vi "LV Exp7.vi"() -> ()   [LabVIEW 2009]
uses:
  <vilib>/NXT/Block Support/NXT_InputPort.ctl
  <vilib>/NXT/Dual Mode Library/Waits/Wait_Num(msec).vi
  <vilib>/NXT/Dual Mode Library/Display/drawText.vi
panel:
  out "Detected":bool
  # "HiTechnic Experimenter's Kit\n\n                        Experiment 7 - Magnetic Switch\nThis program reads the status of the Hall Effect Sensor on B0\nto determine if a magnetic field is presen and if it is present\nthe LED on B4 is truned on.\n\nSee Experimenter's Kit Handbook for the SuperPro for\nmore information or go to www.hitechnic.com. \n\n(c) HiTechnic 2011"
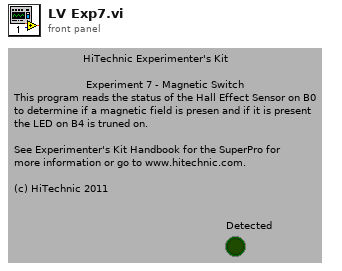
[diagram p1: front panel]
types:
  T1 = typedef "NXT_InputPort.ctl" = u8
  T2 = typedef "LVHSConnector.ctl" = cluster{"error":errorcluster, "address":string, "NXT #":i32, "Show Error":bool, "Connection":u16}
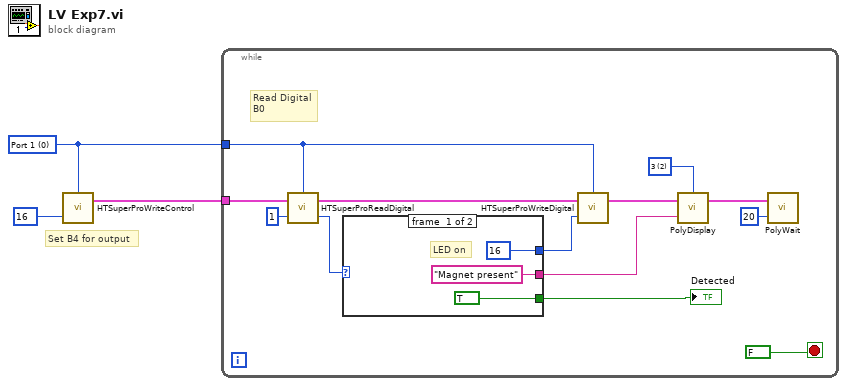
[diagram p0: block diagram]
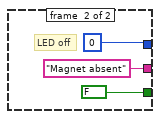
[diagram p2: hidden frame]
diagram:
  w1 = T1 0 items=["Port 1", "Port 2", "Port 3", "Port 4"] ("Port")
  # "Set B4 for output"
  n1 = call "HTSuperProWriteControl.vi"("Digital Value"=u8 16, "Port"=w1) -> ("NXT"=w2:T2)  [unwired: 3 in]
  n2 = while {
    tunnel: w2 -> [w13]
    tunnel: w1 -> [w10]
    stop <- FALSE stop-if-true
    w4 = i16 2 items=["1", "2", "3", "4", "5", "6", "7", "8"] ("Line")
    # "Read Digital\nB0"
    n3 = call "HTSuperProReadDigital.vi"("Mask"=u8 1, "NXT"=w13, "Port"=w10) -> ("Digital Value"=w12:u8, "NXT"=w11:T2)  [unwired: 1 in]
    n4 = case shown="1" w12 {
      tunnel: ["Magnet present" "Magnet absent"] -> w7
      tunnel: [TRUE FALSE] -> w15
      tunnel: [u8 16 u8 0] -> w9
      frame #0 {
        # "LED on"
      }
      frame #1 {
        # "LED off"
      }
    }
    "Detected" <- w15
    n5 = call "HTSuperProWriteDigital.vi"("Digital Value"=w9, "NXT"=w11, "Port"=w10) -> ("NXT"=w8:T2)  [unwired: 2 in]
    n6 = call-poly <vilib>:"PolyDisplay.vi"("Text"=w7, "NXT"=w8, "Line"=w4) -> ("NXT"=w6:T2)  [unwired: 1 in]
    n7 = call-poly <vilib>:"PolyWait.vi"("Time (100 msec)"=u32 20, "NXT"=w6) -> ()  [unwired: 2 in, 1 out]
  }
